vi "Property Dialog.vi"(6 "Control Ref Queue":T15, 7 "Multiplot Representation":T12, 8 "error in (no error)":errorcluster, 11 "2D Error Bar.lvclass in":refnum<class "2D Error Bar.lvclass">) -> (0 "error out":errorcluster, 3 "2D Error Bar.lvclass out":refnum<class "2D Error Bar.lvclass">, 4 "Cancel?":bool)   [LabVIEW 2020, in "2D Error Bar.lvclass"]
uses:
  <vilib>/Math Plots/2D Math Plots/2D Error Bar/2D Error Bar/2D Error Bar.lvclass
  e:/builds/penguin/labview/branches/2020/dev/dist/vi.lib/Math Plots/2D Math Plots/2D Plot/2D Plot/2D Plot.lvclass
  <vilib>/Math Plots/2D Math Plots/2D Plot/Action String/2DMathPlot Ctrl Act Queue.ctl
  <vilib>/Math Plots/2D Math Plots/2D Plot/Action String/2DMathPlot Ctrl Act Cluster.ctl
  <vilib>/Math Plots/2D Math Plots/2D Plot/Action String/2DMathPlot State Class.ctl
  <vilib>/Math Plots/2D Math Plots/2D Plot/2D Plot/Typedef/Multiplot Representation.ctl
  <vilib>/Math Plots/2D Math Plots/2D Plot/2D Plot/Typedef/Plot Representation.ctl
  <vilib>/Math Plots/2D Math Plots/2D Plot/2D Plot/Typedef/Range Cluster.ctl
  <vilib>/Math Plots/2D Math Plots/2D Plot/2D Plot/Typedef/Cursor Property.ctl
  <vilib>/Utility/miscctls.llb/LVCursorListTypeDef.ctl
  <vilib>/Math Plots/2D Math Plots/2D Plot/2D Plot/Typedef/Scale Cluster.ctl
  <vilib>/Utility/miscctls.llb/LVOffsetAndMultiplierTypeDef.ctl
  <vilib>/Math Plots/2D Math Plots/2D Error Bar/2D Error Bar/Typedef/2D Error Bar Property Cluster.ctl
  <vilib>/Math Plots/2D Math Plots/2D Plot/2D Plot/Typedef/Plot Property Array.ctl
  <vilib>/Math Plots/2D Math Plots/2D Plot/2D Plot/Typedef/Plot Property.ctl
  <vilib>/Math Plots/2D Math Plots/2D Error Bar/2D Error Bar/Typedef/2D Error Bar Property Array.ctl
  <vilib>/Math Plots/2D Math Plots/2D Error Bar/2D Error Bar/Typedef/2D Error Bar Property.ctl
  <vilib>/Math Plots/2D Math Plots/2D Plot/2D Plot/Typedef/Graph General Property.ctl
  <vilib>/Math Plots/2D Math Plots/2D Plot/2D Plot/Typedef/Temp Graph Data Action.ctl
  <vilib>/Math Plots/2D Math Plots/2D Plot/2D Plot/Typedef/Temp Graph State.ctl
  <vilib>/Math Plots/2D Math Plots/2D Error Bar/2D Error Bar/2D Error Bar.lvclass/2D Error Bar.ctl
  <vilib>/Math Plots/2D Math Plots/2D Plot/2D Plot/2D Plot.lvclass
panel:
  in  "Graph General":T1
  in  "Format String":string[](array[string])
  in  "Error Bar Property":T2
  in  "Scales Array":T7[](array[typedef])
  in  "Cursor Property":T9
  in  "Dialog Tab":enum32{"UI", "Input & Output"}(tab)
  in  "OK":bool
  in  "Cancel":bool
  in  "Help":bool
  in  "Page Tab":T11(tab)
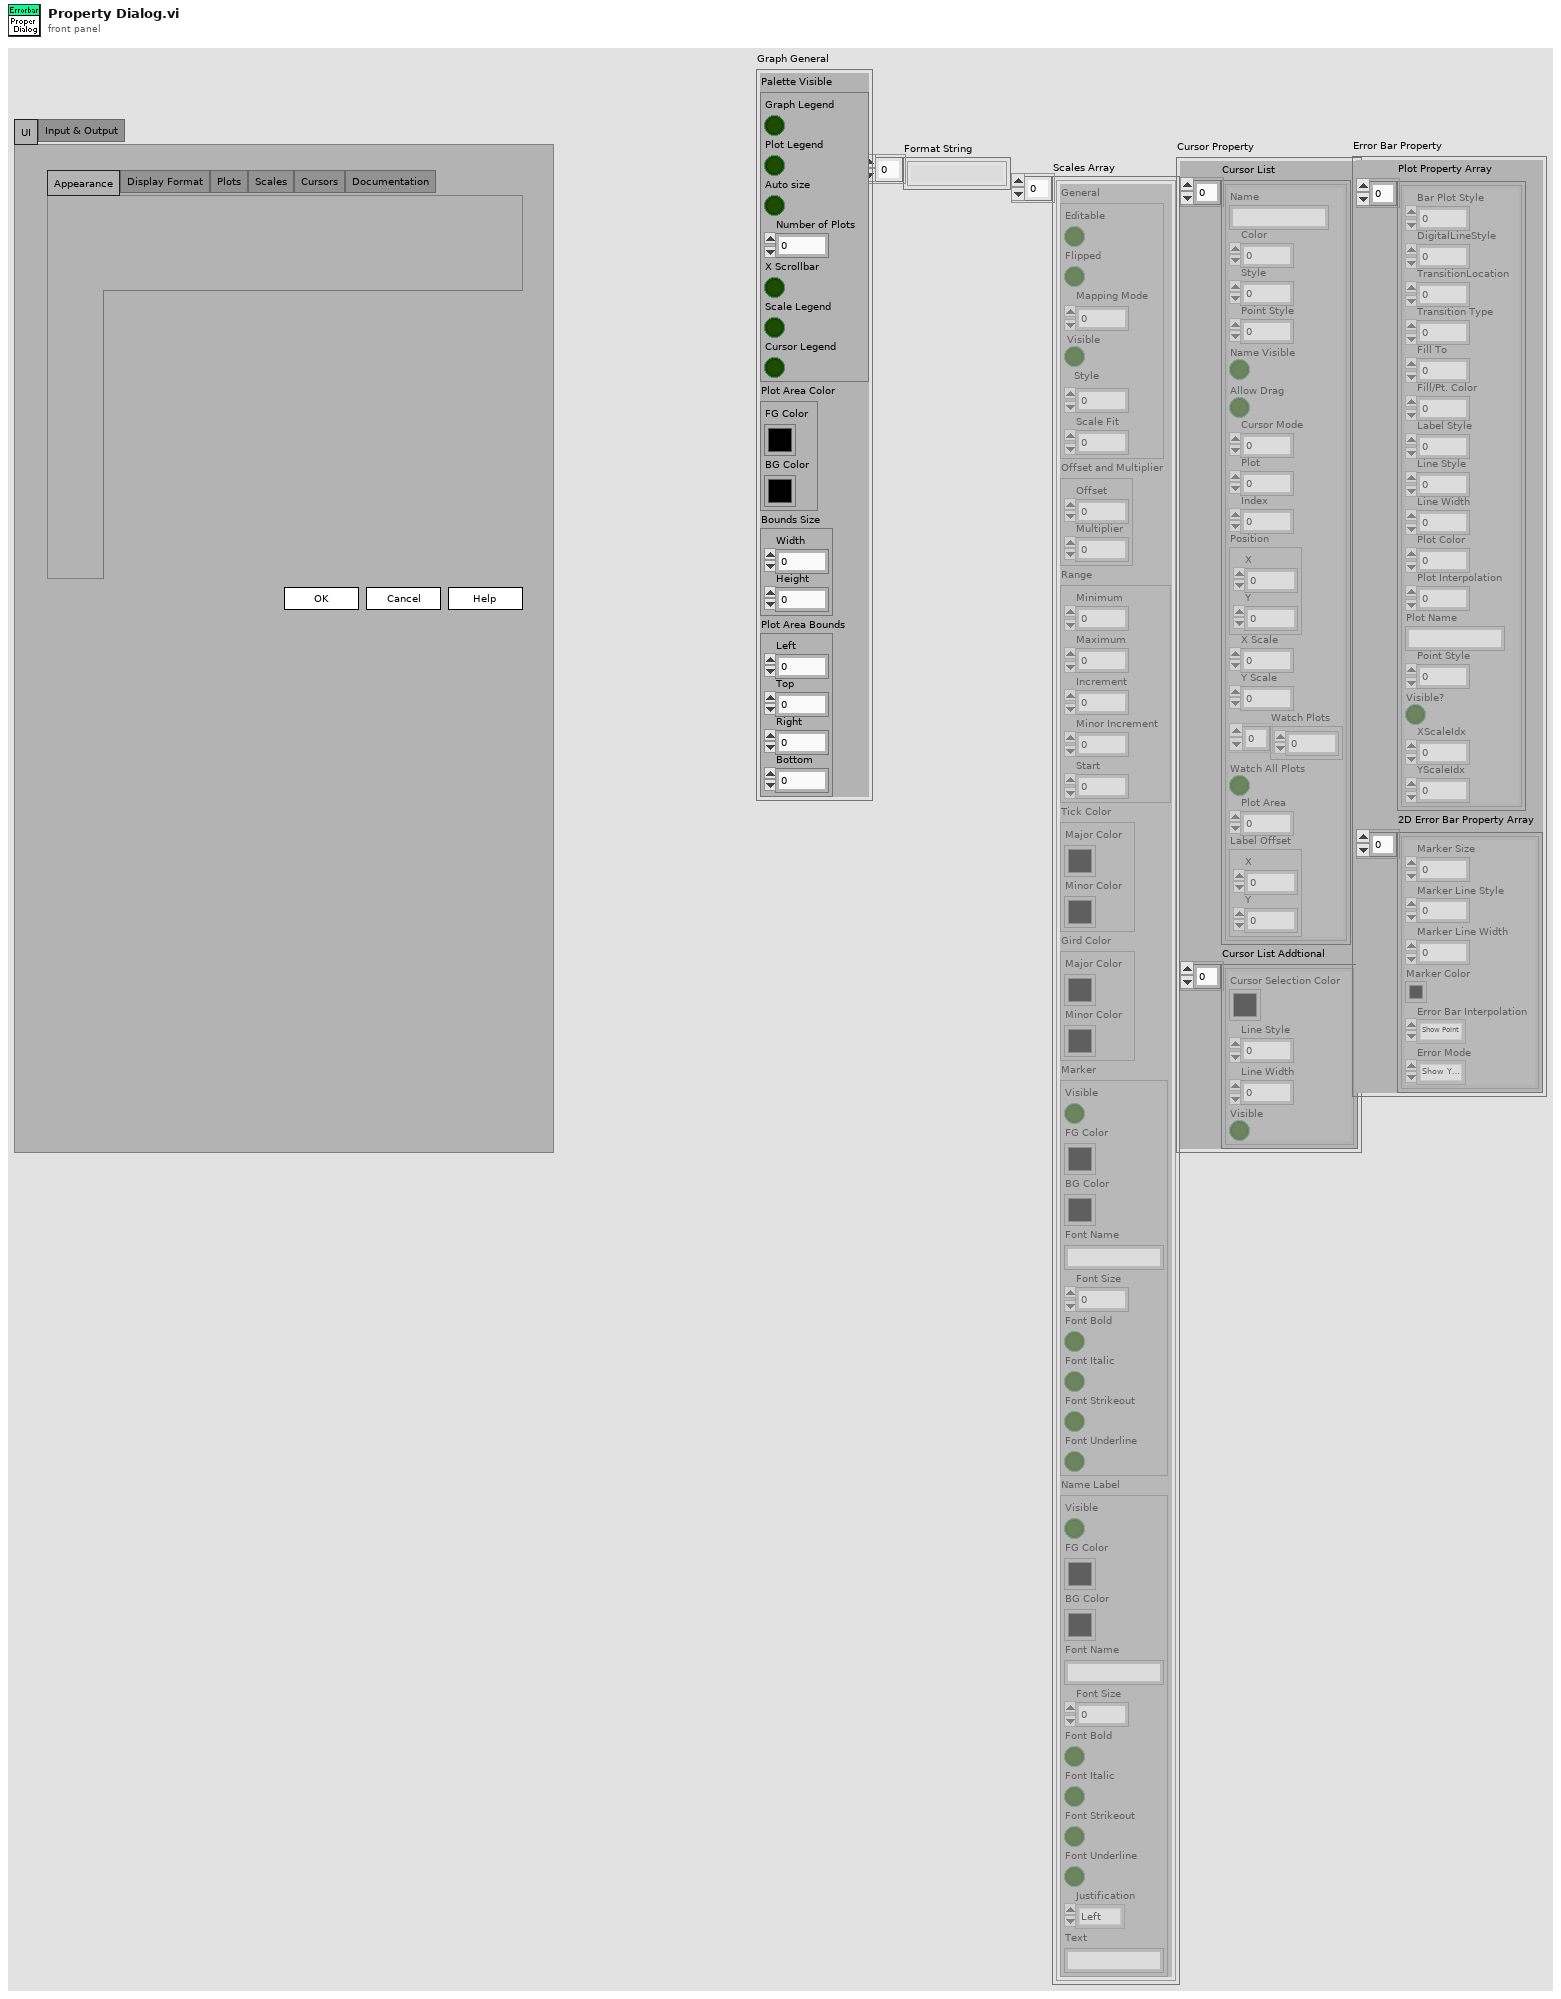
[diagram p1: front panel]
types:
  T1 = typedef "2D Plot.lvclass/Graph General Property.ctl" = cluster{"Palette Visible":cluster{"Graph Legend":bool, "Plot Legend":bool, "Auto size":bool, "Number of Plots":u32, "X Scrollbar":bool, "Scale Legend":bool, "Cursor Legend":bool}, "Plot Area Color":cluster{"FG Color":u32, "BG Color":u32}, "Bounds Size":cluster{"Width":u32, "Height":u32}, "Plot Area Bounds":cluster{"Left":i16, "Top":i16, "Right":i16, "Bottom":i16}}
  T2 = typedef "2D Error Bar.lvclass/2D Error Bar Property Cluster.ctl" = cluster{"Plot Property Array":T3, "2D Error Bar Property Array":T5}
  T3 = typedef "2D Plot.lvclass/Plot Property Array.ctl" = T4[]
  T4 = typedef "2D Plot.lvclass/Plot Property.ctl" = cluster{"Bar Plot Style":u8, "DigitalLineStyle":u8, "TransitionLocation":u8, "Transition Type":u8, "Fill To":i16, "Fill/Pt. Color":u32, "Label Style":u8, "Line Style":u8, "Line Width":u8, "Plot Color":u32, "Plot Interpolation":u8, "Plot Name":string, "Point Style":u8, "Visible?":bool, "XScaleIdx":u32, "YScaleIdx":u32}
  T5 = typedef "2D Error Bar.lvclass/2D Error Bar Property Array.ctl" = T6[]
  T6 = typedef "2D Error Bar.lvclass/2D Error Bar Property.ctl" = cluster{"Marker Size":dbl, "Marker Line Style":u8, "Marker Line Width":u8, "Marker Color":u32, "Error Bar Interpolation":enum16{"Show Point", "Show Line", "Show Bar"}, "Error Mode":enum16{"Show Y Error", "Show X Error", "Show Both Error"}}
  T7 = typedef "2D Plot.lvclass/Scale Cluster.ctl" = cluster{"General":cluster{"Editable":bool, "Flipped":bool, "Mapping Mode":u8, "Visible":bool, "Style":u8, "Scale Fit":u8}, "Offset and Multiplier":T8, "Range":cluster{"Minimum":dbl, "Maximum":dbl, "Increment":dbl, "Minor Increment":dbl, "Start":dbl}, "Tick Color":cluster{"Major Color":u32, "Minor Color":u32}, "Gird Color":cluster{"Major Color":u32, "Minor Color":u32}, "Marker":cluster{"Visible":bool, "FG Color":u32, "BG Color":u32, "Font Name":string, "Font Size":u32, "Font Bold":bool, "Font Italic":bool, "Font Strikeout":bool, "Font Underline":bool}, "Name Label":cluster{"Visible":bool, "FG Color":u32, "BG Color":u32, "Font Name":string, "Font Size":u32, "Font Bold":bool, "Font Italic":bool, "Font Strikeout":bool, "Font Underline":bool, "Justification":enum16{"Left", "Center", "Right"}, "Text":string}}
  T8 = typedef "LVOffsetAndMultiplierTypeDef.ctl" = cluster{"Offset":dbl, "Multiplier":dbl}
  T9 = typedef "2D Plot.lvclass/Cursor Property.ctl" = cluster{"Cursor List":T10, "Cursor List Addtional":cluster{"Cursor Selection Color":u32, "Line Style":u8, "Line Width":u8, "Visible":bool}[]}
  T10 = typedef "LVCursorListTypeDef.ctl" = cluster{"Name":string, "Color":u32, "Style":u8, "Point Style":u8, "Name Visible":bool, "Allow Drag":bool, "Cursor Mode":u32, "Plot":i32, "Index":i32, "Position":cluster{"X":dbl, "Y":dbl}, "X Scale":u32, "Y Scale":u32, "Watch Plots":i32[], "Watch All Plots":bool, "Plot Area":i32, "Label Offset":cluster{"X":dbl, "Y":dbl}}[]
  T11 = enum32{"Appearance", "Display Format", "Plots", "Scales", "Cursors", "Documentation"}
  T12 = typedef "2D Plot.lvclass/Multiplot Representation.ctl" = cluster{"Plot Representation Array":T13[], "Max Range":T14}
  T13 = typedef "2D Plot.lvclass/Plot Representation.ctl" = cluster{"Plot Range":T14, "Vertex Cluster":cluster{"Vertex X Array":dbl[], "Vertex Y Array":dbl[]}, "Base Cluster":cluster{"Base X Array":dbl[], "Base Y Array":dbl[]}}
  T14 = typedef "2D Plot.lvclass/Range Cluster.ctl" = cluster{"X Range":cluster{"Max X":dbl, "Min X":dbl}, "Y Range":cluster{"Max Y":dbl, "Min Y":dbl}}
  T15 = typedef "2DMathPlot Ctrl Act Queue.ctl" = refnum<queue>
  T16 = typedef "2D Plot.lvclass/Temp Graph State.ctl" = enum16{"Create", "Update Graph", "Update Property Only", "Get Plot Name", "Get Axis Name", "Destory"}
  T17 = typedef "2D Plot.lvclass/Temp Graph Data Action.ctl" = enum16{"Data Cluster", "Property Class", "Control Queue"}
  T18 = typedef "2D Plot.lvclass/Property Cluster.ctl" = cluster{"Graph General":T1, "Format Property":string[], "Scale Array":T19, "Cursor Property":T9, "Annotation List":T20, "Active Cursor":i32, "Active Plot":i32}
  T19 = typedef "2D Plot.lvclass/Scale Array.ctl" = T7[]
  T20 = typedef "LVAnnotationListTypeDef.ctl" = cluster{"Name":string, "Color":u32, "Style":u8, "Point Style":u8, "Name Visible":bool, "Allow Drag":bool, "Annotation Mode":u32, "Plot":i32, "Index":i32, "Position":cluster{"X":dbl, "Y":dbl}, "X Scale":u32, "Y Scale":u32, "Show Arrow":bool, "Lock Name":bool, "Plot Area":i32, "Label Offset":cluster{"X":dbl, "Y":dbl}}[]
  T21 = typedef "2DMathPlot Ctrl Act Cluster.ctl" = cluster{"Plot Area Ref":refnum<vi>, "Z Axis Ref":refnum<vi>, "Legend Ref":refnum<vi>, "XControl Ref":refnum<vi>, "Facade Ref":refnum<vi>, "Display State Change Class":T22}
  T22 = typedef "2DMathPlot State Class.ctl" = enum16{"Update All (Undo)", "Update General", "Update Appearance", "Update Format", "Update Scale", "Update Marker", "Update Cursor", "None"}
  T23 = enum8{"Enabled", "Disabled", "Disabled and Grayed Out"}
  T24 = enum32{"Bad", "Idle", "Run top level", "Running"}[]
  T25 = enum32{"Bad", "Idle", "Run top level", "Running"}
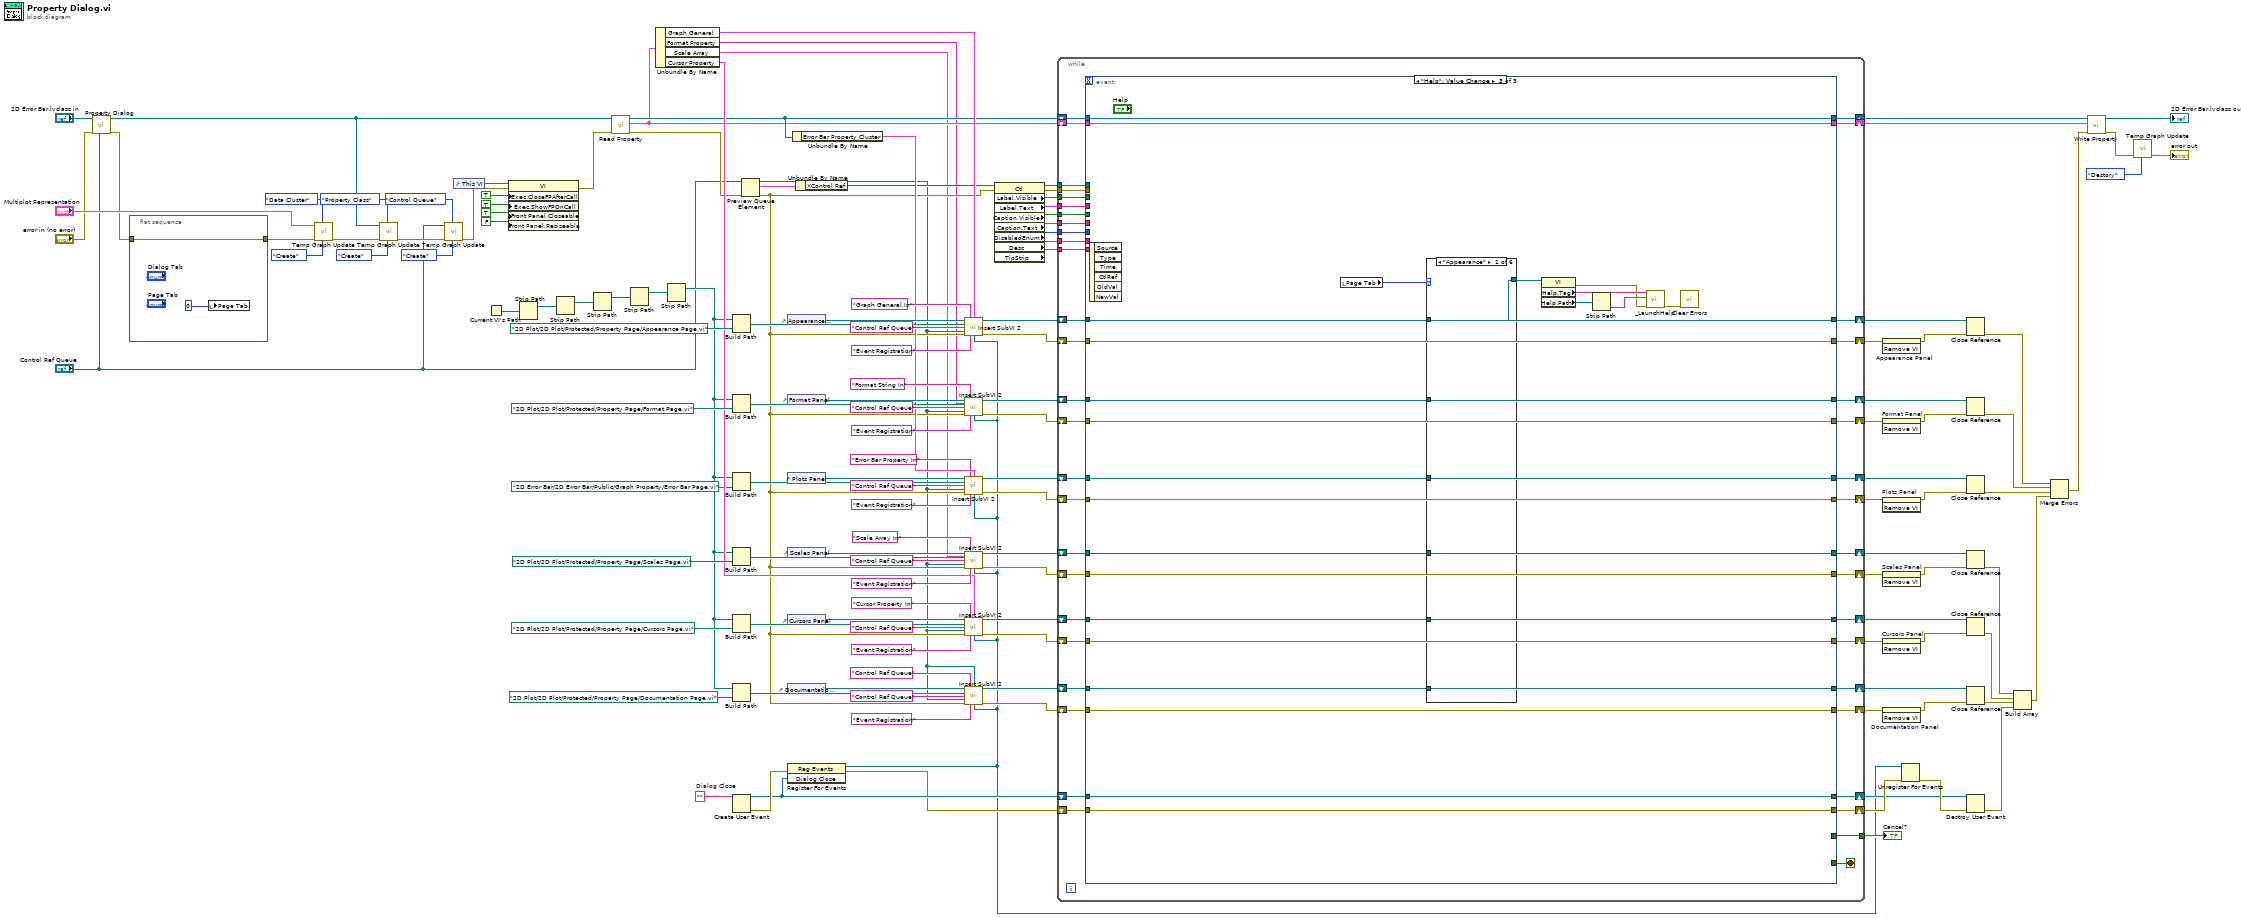
[diagram p0: block diagram]
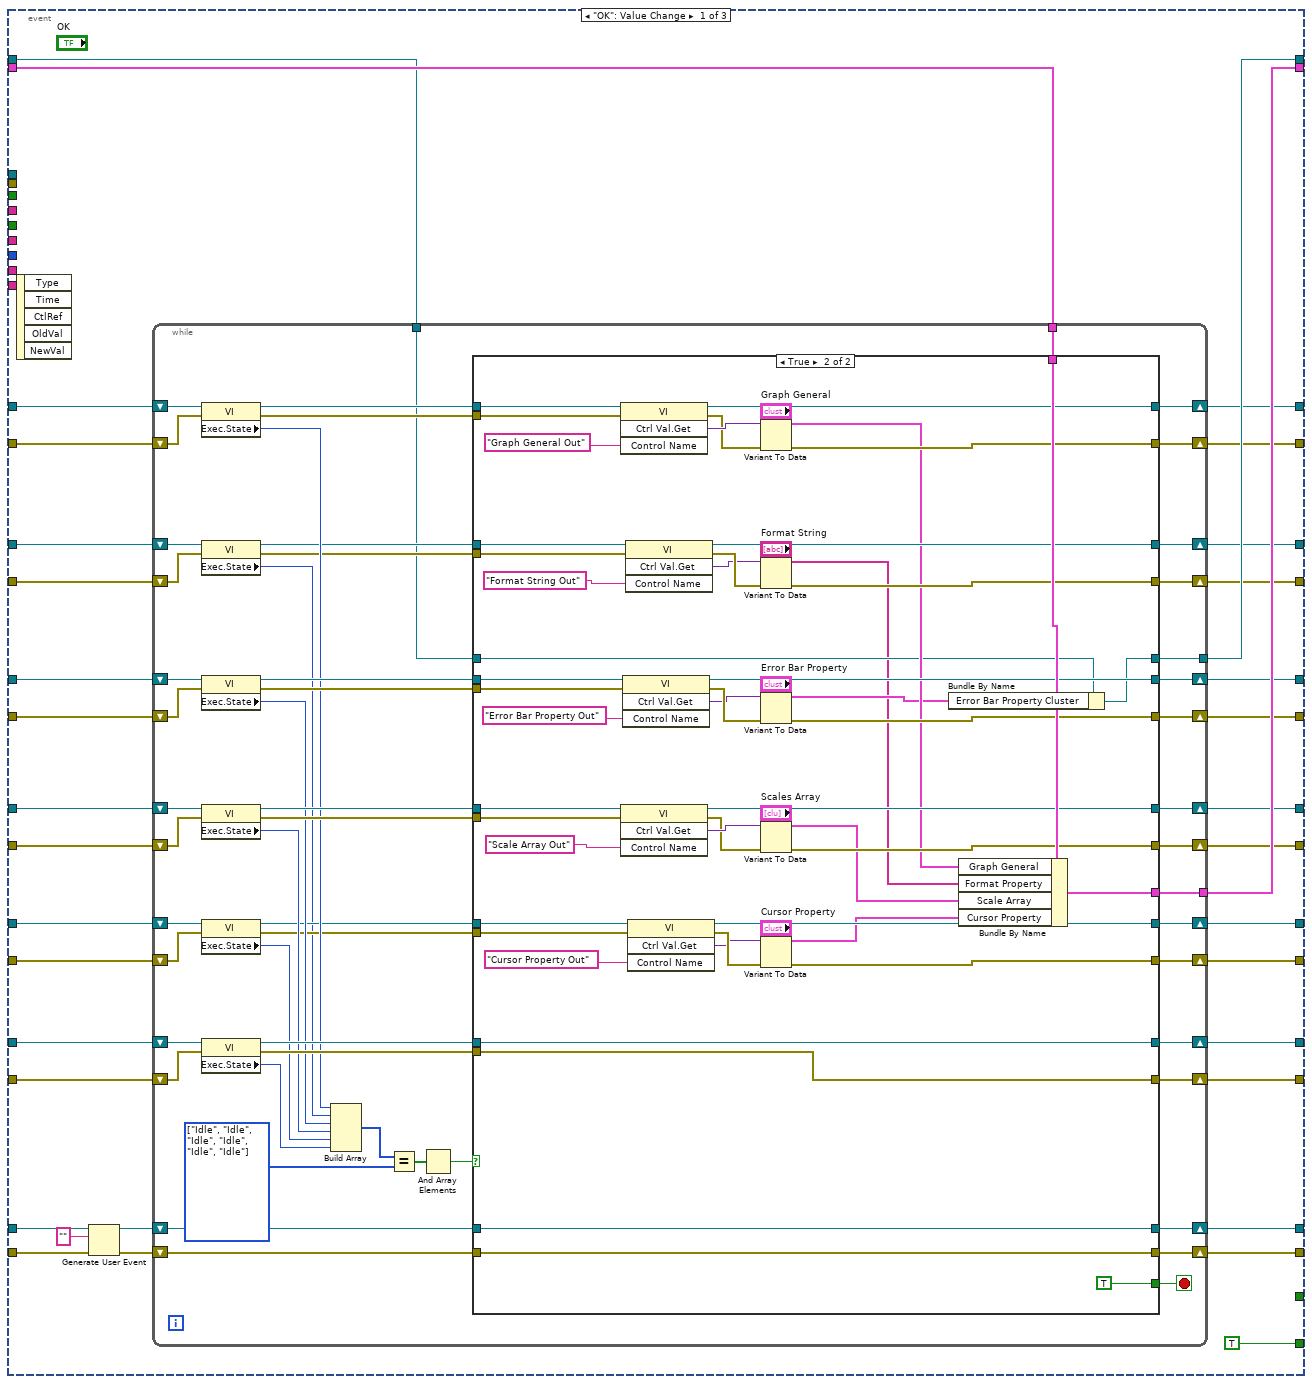
[diagram p2: hidden frame]
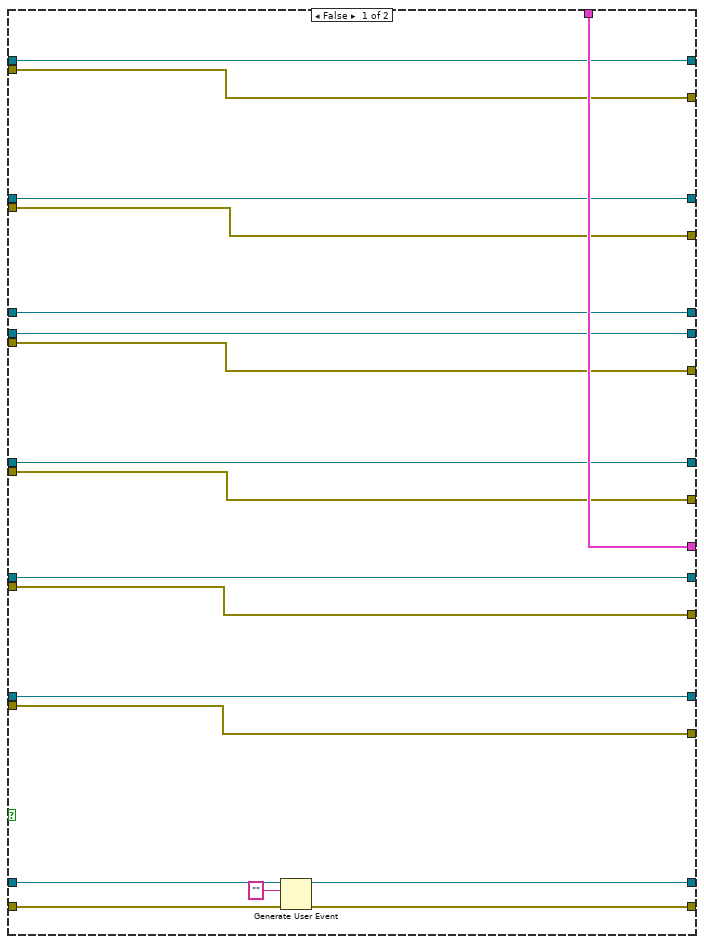
[diagram p3: hidden frame]
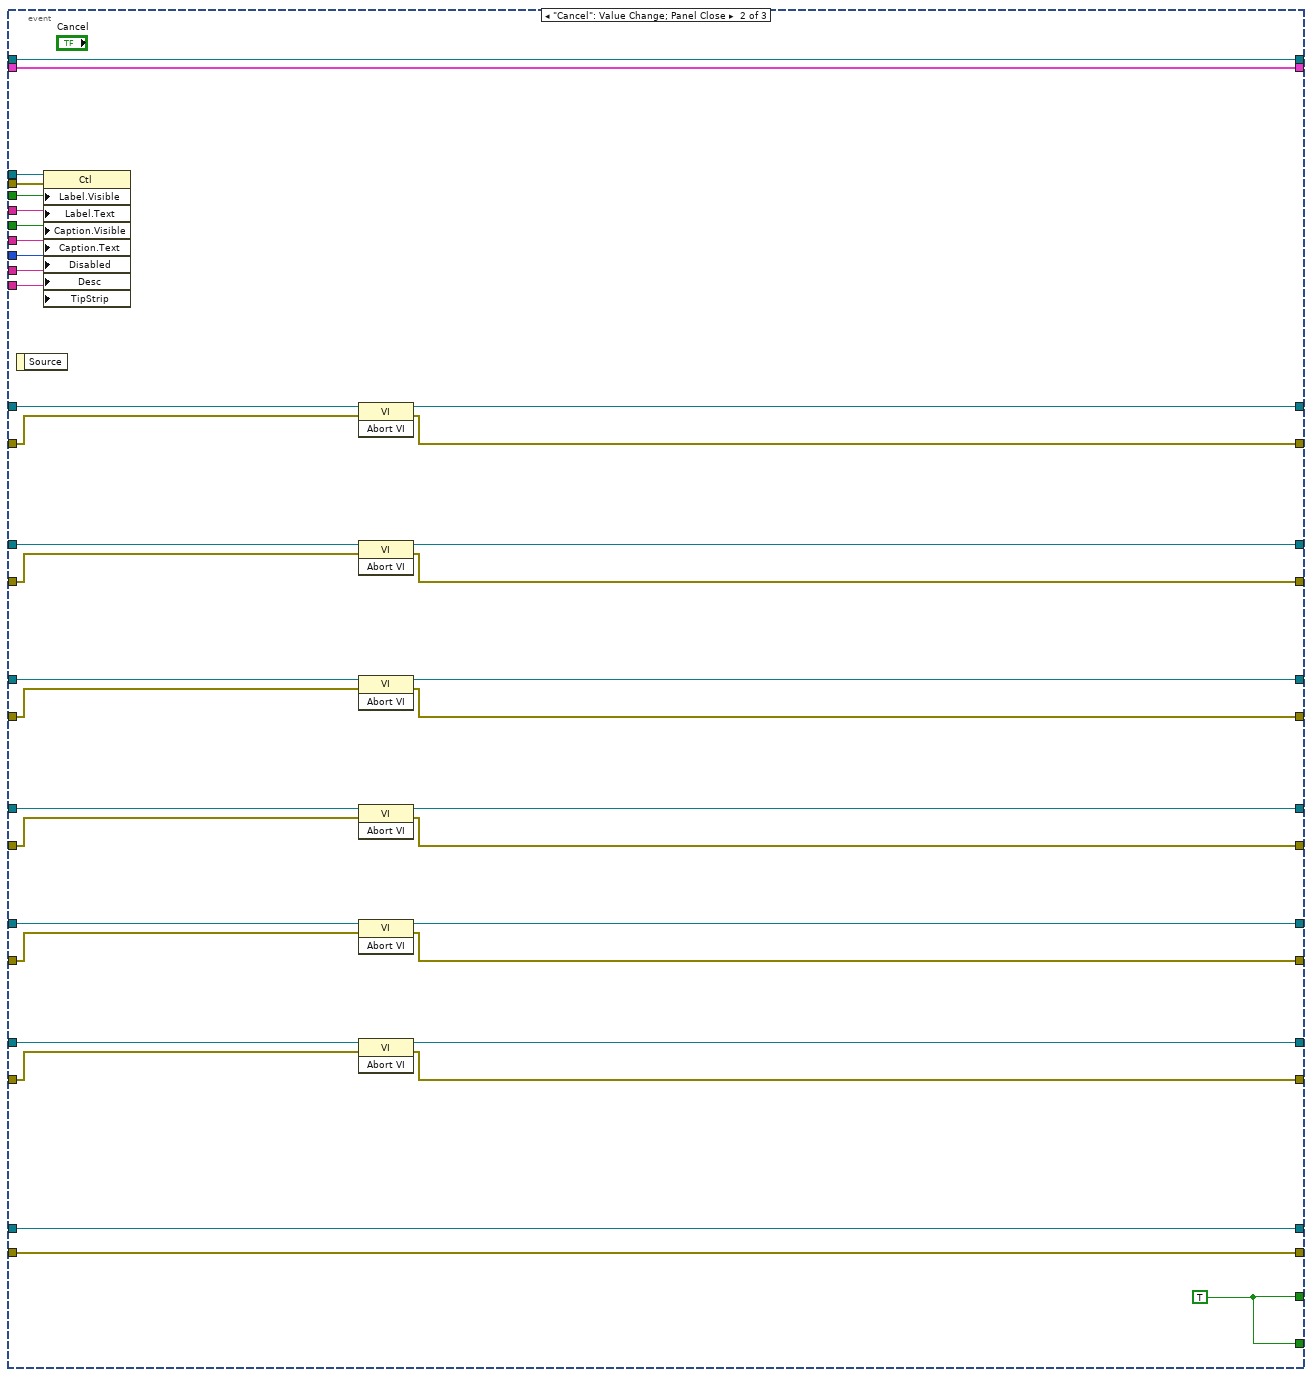
[diagram p4: hidden frame]
diagram:
  w122 = ""  # Dialog Close
  n1 = call-parent "Property Dialog.vi"("Control Ref Queue"="Control Ref Queue", "error in (no error)"="error in (no error)", "2D Plot.lvclass in"="2D Error Bar.lvclass in") -> ("error out"=w2:errorcluster, "2D Plot.lvclass out"=w4:refnum<class "2D Error Bar.lvclass">)  [unwired: 1 in, 6 out]
  n2 = flat-sequence {
    tunnel: w2 -> [w140]
    tunnel: [w140] -> w27
    frame #0 {
      n3 = local write "Page Tab"(u32 0) -> ()
    }
  }
  n4 = call <vilib>:"Temp Graph Update.vi"("State"=Temp_Graph_State."Create", "Data Name"=Temp_Graph_Data_Action."Data Cluster", "error in (no error)"=w27, "Property In"="Multiplot Representation") -> ("error out"=w26:errorcluster)  [unwired: 1 in, 6 out]
  n5 = call <vilib>:"Temp Graph Update.vi"("State"=Temp_Graph_State."Create", "Data Name"=Temp_Graph_Data_Action."Property Class", "error in (no error)"=w26, "Property In"=w4) -> ("error out"=w25:errorcluster)  [unwired: 1 in, 6 out]
  n6 = call <vilib>:"Temp Graph Update.vi"("State"=Temp_Graph_State."Create", "Data Name"=Temp_Graph_Data_Action."Control Queue", "error in (no error)"=w25, "Property In"="Control Ref Queue") -> ("error out"=w18:errorcluster)  [unwired: 1 in, 6 out]
  n7 = control-ref of="This VI"() -> (w139:refnum<vi>)
  n8 = Current VI's Path() -> (path=w131:path)
  n9 = property class="VI"(reference=w139, error in=w18, "Exec.CloseFPAfterCall"=TRUE ("Execution:Close After Call"), "Exec.ShowFPOnCall"=TRUE ("Execution:Show Front Panel On Call"), "Front Panel.Closeable"=TRUE ("Front Panel Window:Closeable"), "Front Panel.Resizeable"=FALSE ("Front Panel Window:Resizeable")) -> (error out=w129:errorcluster)  [unwired: 1 out]
  n10 = Strip Path(path=w131) -> (stripped path=w132:path)  [unwired: 1 out]
  n11 = Strip Path(path=w132) -> (stripped path=w133:path)  [unwired: 1 out]
  n12 = Strip Path(path=w133) -> (stripped path=w130:path)  [unwired: 1 out]
  n13 = call <vilib>:"Read Property.vi"("error in (no error)"=w129, "2D Plot.lvclass in"=w4) -> ("error out"=w39:errorcluster, "XY Graph Property Cluster"=w87:T18, "2D Plot.lvclass out"=w88:refnum<class "2D Error Bar.lvclass">)  [unwired: 7 out]
  n14 = Strip Path(path=w130) -> (stripped path=w7:path)  [unwired: 1 out]
  n15 = Unbundle By Name(w87) -> ("Graph General"=w125:T1, "Format Property"=w9:string[], "Scale Array"=w8:T19, "Cursor Property"=w107:T9)
  n16 = Strip Path(path=w7) -> (stripped path=w6:path)  [unwired: 1 out]
  n17 = Build Path(base path=w6, name or relative path=path "2D Plot/2D Plot/Protected/Property Page/Appearance Page.vi") -> (appended path=w128:path)
  n18 = Build Path(base path=w6, name or relative path=path "2D Plot/2D Plot/Protected/Property Page/Format Page.vi") -> (appended path=w118:path)
  n19 = Build Path(base path=w6, name or relative path=path "2D Error Bar/2D Error Bar/Public/Graph Property/Error Bar Page.vi") -> (appended path=w91:path)
  n20 = Build Path(base path=w6, name or relative path=path "2D Plot/2D Plot/Protected/Property Page/Scales Page.vi") -> (appended path=w112:path)
  n21 = Build Path(base path=w6, name or relative path=path "2D Plot/2D Plot/Protected/Property Page/Cursors Page.vi") -> (appended path=w102:path)
  n22 = Build Path(base path=w6, name or relative path=path "2D Plot/2D Plot/Protected/Property Page/Documentation Page.vi") -> (appended path=w93:path)
  n23 = Create User Event(user event datatype=w122) -> (user event=w74:refnum<user-event>, error out=w123:errorcluster)  [unwired: 1 in]
  n24 = Preview Queue Element(queue="Control Ref Queue", error in (no error)=w39) -> (queue out=w12:T15, element=w38:T21, error out=w13:errorcluster)  [unwired: 2 out]
  n25 = control-ref of="Appearance Panel"() -> (w127:refnum<vi>)
  n26 = control-ref of="Format Panel"() -> (w119:refnum<vi>)
  n27 = control-ref of="Plots Panel"() -> (w98:refnum<vi>)
  n28 = control-ref of="Scales Panel"() -> (w114:refnum<vi>)
  n29 = control-ref of="Cursors Panel"() -> (w104:refnum<vi>)
  n30 = control-ref of="Documentation Panel"() -> (w101:refnum<vi>)
  n31 = register-events(error in=w123, w74) -> (reference out=w11:refnum<event-registration>, error out=w73:errorcluster)  [unwired: 1 in]
  n32 = Unbundle By Name(w88) -> ("Error Bar Property Cluster"=w95:T2)
  n33 = Unbundle By Name(w38) -> ("XControl Ref"=w37:refnum<vi>)
  n34 = call <vilib>:"Insert SubVI 2.vi"("Sub Panel Ref"=w127, "Label 1"="Graph General In", "Value 1"=w125, "VI Path"=w128, "Label 3"="Control Ref Queue" ("Label 1"), "Value 3"=w12, "error in (no error)"=w13, "Label 2"="Event Registration", "Value 2"=w11) -> ("vi reference"=w86:refnum<vi>, "error out"=w80:errorcluster)  [unwired: 5 out]
  n35 = call <vilib>:"Insert SubVI 2.vi"("Sub Panel Ref"=w119, "Label 1"="Format String In" ("Label 2"), "Value 1"=w9, "VI Path"=w118, "Label 3"="Control Ref Queue" ("Label 1"), "Value 3"=w12, "error in (no error)"=w13, "Label 2"="Event Registration", "Value 2"=w11) -> ("vi reference"=w85:refnum<vi>, "error out"=w79:errorcluster)  [unwired: 5 out]
  n36 = call <vilib>:"Insert SubVI 2.vi"("Sub Panel Ref"=w98, "Label 1"="Error Bar Property In", "Value 1"=w95, "VI Path"=w91, "Label 3"="Control Ref Queue" ("Label 1"), "Value 3"=w12, "error in (no error)"=w13, "Label 2"="Event Registration", "Value 2"=w11) -> ("vi reference"=w84:refnum<vi>, "error out"=w78:errorcluster)  [unwired: 5 out]
  n37 = call <vilib>:"Insert SubVI 2.vi"("Sub Panel Ref"=w114, "Label 1"="Scale Array In", "Value 1"=w8, "VI Path"=w112, "Label 3"="Control Ref Queue" ("Label 1"), "Value 3"=w12, "error in (no error)"=w13, "Label 2"="Event Registration", "Value 2"=w11) -> ("vi reference"=w83:refnum<vi>, "error out"=w77:errorcluster)  [unwired: 5 out]
  n38 = call <vilib>:"Insert SubVI 2.vi"("Sub Panel Ref"=w104, "Label 1"="Cursor Property In", "Value 1"=w107, "VI Path"=w102, "Label 3"="Control Ref Queue" ("Label 1"), "Value 3"=w12, "error in (no error)"=w13, "Label 2"="Event Registration", "Value 2"=w11) -> ("vi reference"=w82:refnum<vi>, "error out"=w76:errorcluster)  [unwired: 5 out]
  n39 = call <vilib>:"Insert SubVI 2.vi"("Sub Panel Ref"=w101, "Label 1"="Control Ref Queue", "Value 1"=w12, "VI Path"=w93, "Label 3"="Control Ref Queue" ("Label 1"), "Value 3"=w12, "error in (no error)"=w13, "Label 2"="Event Registration", "Value 2"=w11) -> ("vi reference"=w81:refnum<vi>, "error out"=w75:errorcluster)  [unwired: 5 out]
  n40 = property class="Ctl"(reference=w37, error in=w13) -> (reference out=w36:refnum<vi>, error out=w35:errorcluster, "Label.Visible"=w34:bool, "Label.Text"=w33:string, "Caption.Visible"=w32:bool, "Caption.Text"=w31:string, "DisabledEnum"=w30:T23, "Desc"=w29:string, "TipStrip"=w28:string)
  n41 = while {
    shift-right: [w168] -> w70
    shift-left: w88 -> [w184]
    shift-right: [w167] -> w71
    shift-left: w87 -> [w183]
    shift-right: [w166] -> w61
    shift-left: w80 -> [w176]
    shift-right: [w165] -> w59
    shift-left: w79 -> [w175]
    shift-right: [w164] -> w53
    shift-left: w78 -> [w174]
    shift-right: [w163] -> w50
    shift-left: w77 -> [w173]
    shift-right: [w162] -> w49
    shift-left: w76 -> [w172]
    shift-right: [w161] -> w45
    shift-left: w75 -> [w171]
    shift-right: [w160] -> w42
    shift-left: w73 -> [w169]
    shift-right: [w153] -> w40
    shift-left: w74 -> [w170]
    shift-right: [w154] -> w44
    shift-left: w81 -> [w177]
    shift-right: [w155] -> w48
    shift-left: w82 -> [w178]
    shift-right: [w156] -> w52
    shift-left: w83 -> [w179]
    shift-right: [w157] -> w54
    shift-left: w84 -> [w180]
    shift-right: [w158] -> w57
    shift-left: w85 -> [w181]
    shift-right: [w159] -> w62
    shift-left: w86 -> [w182]
    tunnel: [w151] -> w72
    tunnel: w36 -> [w150]
    tunnel: w35 -> [w149]
    tunnel: w34 -> [w148]
    tunnel: w33 -> [w147]
    tunnel: w32 -> [w146]
    tunnel: w31 -> [w145]
    tunnel: w30 -> [w144]
    tunnel: w29 -> [w143]
    tunnel: w28 -> [w142]
    stop <- w152 stop-if-true
    n42 = event shown="[2] \"Help\": Value Change" {
      selector: _ -> [_ _ _]
      dyn-events: _ -> [_ _ _]
      timeout: _ -> [_ _ _]
      tunnel: w184 -> [w202 w359 w400]
      tunnel: w183 -> [w203 w360 w401]
      tunnel: w182 -> [w220 w386 w392]
      tunnel: w181 -> [w219 w382 w391]
      tunnel: w180 -> [w218 w380 w390]
      tunnel: w179 -> [w217 w378 w389]
      tunnel: w178 -> [w216 w376 w388]
      tunnel: w177 -> [w215 w374 w387]
      tunnel: w176 -> [w214 w385 w409]
      tunnel: w175 -> [w213 w381 w408]
      tunnel: w174 -> [w212 w379 w407]
      tunnel: w173 -> [w211 w377 w406]
      tunnel: w172 -> [w210 w375 w405]
      tunnel: w171 -> [w209 w373 w404]
      tunnel: w170 -> [w205 w362 w402]
      tunnel: w169 -> [w206 w361 w403]
      tunnel: [w201 w359 w400] -> w168
      tunnel: [w200 w360 w401] -> w167
      tunnel: [w199 w383 w409] -> w166
      tunnel: [w198 w371 w408] -> w165
      tunnel: [w185 w369 w407] -> w164
      tunnel: [w186 w367 w406] -> w163
      tunnel: [w197 w365 w405] -> w162
      tunnel: [w196 w363 w404] -> w161
      tunnel: [w195 w361 w403] -> w160
      tunnel: [w194 w384 w392] -> w159
      tunnel: [w193 w372 w391] -> w158
      tunnel: [w192 w370 w390] -> w157
      tunnel: [w191 w368 w389] -> w156
      tunnel: [w190 w366 w388] -> w155
      tunnel: [w189 w364 w387] -> w154
      tunnel: [w187 w362 w402] -> w153
      tunnel: [TRUE w349 _] -> w152
      tunnel: [_ w349 _] -> w151
      tunnel: w150 -> [_ w358 _]
      tunnel: w149 -> [_ w357 _]
      tunnel: w148 -> [_ w356 _]
      tunnel: w147 -> [_ w355 _]
      tunnel: w146 -> [_ w354 _]
      tunnel: w145 -> [_ w353 _]
      tunnel: w144 -> [_ w352 _]
      tunnel: w143 -> [_ w351 _]
      tunnel: w142 -> [_ w350 _]
      event "OK": Value Change {
        n43 = event-data() -> ()  [unwired: 6 out]
        n44 = Generate User Event(user event=w205, event data cluster="" ("event data"), error in=w206) -> (user event out=w204:refnum<user-event>, error out=w207:errorcluster)  [unwired: 1 in]
        n45 = while {
          tunnel: w203 -> [w275]
          tunnel: [w274] -> w200
          shift-right: [w241] -> w187
          shift-left: w204 -> [w242]
          shift-right: [w225] -> w195
          shift-left: w207 -> [w234]
          tunnel: w202 -> [w224]
          tunnel: [w223] -> w201
          shift-right: [w252] -> w196
          shift-left: w209 -> [w248]
          shift-right: [w251] -> w189
          shift-left: w215 -> [w247]
          shift-right: [w228] -> w190
          shift-left: w216 -> [w233]
          shift-right: [w229] -> w197
          shift-left: w210 -> [w232]
          shift-right: [w222] -> w186
          shift-left: w211 -> [w256]
          shift-right: [w253] -> w191
          shift-left: w217 -> [w257]
          shift-right: [w259] -> w192
          shift-left: w218 -> [w262]
          shift-right: [w221] -> w185
          shift-left: w212 -> [w258]
          shift-right: [w236] -> w193
          shift-left: w219 -> [w239]
          shift-right: [w235] -> w198
          shift-left: w213 -> [w240]
          shift-right: [w273] -> w194
          shift-left: w220 -> [w271]
          shift-right: [w272] -> w199
          shift-left: w214 -> [w269]
          stop <- w263 stop-if-true
          w266 = T24 [enum."Idle", enum."Idle", enum."Idle", enum."Idle", enum."Idle", enum."Idle"] items=["Bad", "Idle", "Run top level", "Running"]
          n46 = property class="VI"(reference=w271, error in=w269) -> (reference out=w270:refnum<vi>, error out=w268:errorcluster, "Exec.State"=w246:T25)
          n47 = property class="VI"(reference=w239, error in=w240) -> (reference out=w238:refnum<vi>, error out=w237:errorcluster, "Exec.State"=w227:T25)
          n48 = property class="VI"(reference=w262, error in=w258) -> (reference out=w261:refnum<vi>, error out=w260:errorcluster, "Exec.State"=w245:T25)
          n49 = property class="VI"(reference=w257, error in=w256) -> (reference out=w255:refnum<vi>, error out=w254:errorcluster, "Exec.State"=w244:T25)
          n50 = property class="VI"(reference=w233, error in=w232) -> (reference out=w231:refnum<vi>, error out=w230:errorcluster, "Exec.State"=w226:T25)
          n51 = property class="VI"(reference=w247, error in=w248) -> (reference out=w249:refnum<vi>, error out=w250:errorcluster, "Exec.State"=w243:T25)
          n52 = Build Array(w246, w227, w245, w244, w226, w243) -> (w267:T24)
          n53 = Equal?(x=w267, y=w266) -> (x = y?=w265:bool[])
          n54 = And Array Elements(Boolean array=w265) -> (logical AND=w264:bool)
          n55 = case shown="True" w264 {
            tunnel: w275 -> [w294 w348]
            tunnel: [w294 w347] -> w274
            tunnel: [w293 w343] -> w273
            tunnel: [w292 w342] -> w272
            tunnel: w270 -> [w293 w341]
            tunnel: w268 -> [w292 w340]
            tunnel: [_ TRUE] -> w263
            tunnel: w261 -> [w290 w334]
            tunnel: w260 -> [w291 w335]
            tunnel: [w291 w333] -> w221
            tunnel: [w290 w332] -> w259
            tunnel: w255 -> [w288 w328]
            tunnel: w254 -> [w289 w327]
            tunnel: [w288 w326] -> w253
            tunnel: [w289 w325] -> w222
            tunnel: w249 -> [w287 w298]
            tunnel: w250 -> [w286 w297]
            tunnel: [w287 w298] -> w251
            tunnel: [w286 w297] -> w252
            tunnel: w242 -> [w285 w324]
            tunnel: [w284 w324] -> w241
            tunnel: w238 -> [w282 w320]
            tunnel: w237 -> [w281 w319]
            tunnel: [w282 w318] -> w236
            tunnel: [w281 w317] -> w235
            tunnel: w234 -> [w280 w316]
            tunnel: [w279 w316] -> w225
            tunnel: w231 -> [w278 w312]
            tunnel: w230 -> [w277 w311]
            tunnel: [w277 w310] -> w229
            tunnel: [w278 w309] -> w228
            tunnel: w224 -> [w276 w305]
            tunnel: [w276 w299] -> w223
            frame False {
              n56 = Generate User Event(user event=w285, event data cluster="" ("event data"), error in=w280) -> (user event out=w284:refnum<user-event>, error out=w279:errorcluster)  [unwired: 1 in]
            }
            frame True {
              n57 = invoke class="VI" method="Ctrl Val.Get"(reference=w341, error in=w340, "Control Name"="Graph General Out") -> (reference out=w343:refnum<vi>, error out=w344:errorcluster, "Get Control Value Variant"=w345:variant)  [unwired: 1 in, 1 out]
              n58 = invoke class="VI" method="Ctrl Val.Get"(reference=w328, error in=w327, "Control Name"="Scale Array Out") -> (reference out=w326:refnum<vi>, error out=w329:errorcluster, "Get Control Value Variant"=w330:variant)  [unwired: 1 in, 1 out]
              n59 = invoke class="VI" method="Ctrl Val.Get"(reference=w334, error in=w335, "Control Name"="Error Bar Property Out") -> (reference out=w332:refnum<vi>, error out=w338:errorcluster, "Get Control Value Variant"=w337:variant)  [unwired: 1 in, 1 out]
              n60 = invoke class="VI" method="Ctrl Val.Get"(reference=w320, error in=w319, "Control Name"="Format String Out") -> (reference out=w318:refnum<vi>, error out=w323:errorcluster, "Get Control Value Variant"=w322:variant)  [unwired: 1 in, 1 out]
              n61 = invoke class="VI" method="Ctrl Val.Get"(reference=w312, error in=w311, "Control Name"="Cursor Property Out") -> (reference out=w309:refnum<vi>, error out=w315:errorcluster, "Get Control Value Variant"=w314:variant)  [unwired: 1 in, 1 out]
              n62 = Variant To Data(error in=w344, type="Graph General", Variant=w345) -> (data=w307:T1, error out=w342:errorcluster)
              n63 = Variant To Data(error in=w323, type="Format String", Variant=w322) -> (data=w295:string[], error out=w317:errorcluster)
              n64 = Variant To Data(error in=w338, type="Error Bar Property", Variant=w337) -> (data=w303:T2, error out=w333:errorcluster)
              n65 = Variant To Data(error in=w329, type="Scales Array", Variant=w330) -> (data=w296:T7[], error out=w325:errorcluster)
              n66 = Variant To Data(error in=w315, type="Cursor Property", Variant=w314) -> (data=w300:T9, error out=w310:errorcluster)
              n67 = Bundle By Name(cluster=w305, "Error Bar Property Cluster"=w303) -> (w299:refnum<class "2D Error Bar.lvclass">)
              n68 = Bundle By Name(cluster=w348, "Graph General"=w307, "Format Property"=w295, "Scale Array"=w296, "Cursor Property"=w300) -> (w347:T18)
            }
          }
        }
      }
      event "Cancel": Value Change; Panel Close {
        w349 = TRUE
        n69 = event-data() -> ()  [unwired: 2 out]
        n70 = property class="Ctl"(reference=w358, error in=w357, "Label.Visible"=w356, "Label.Text"=w355, "Caption.Visible"=w354, "Caption.Text"=w353, "Disabled"=w352, "Desc"=w351, "TipStrip"=w350) -> ()  [unwired: 2 out]
        n71 = invoke class="VI" method="Abort VI"(reference=w386, error in=w385) -> (reference out=w384:refnum<vi>, error out=w383:errorcluster)  [unwired: 1 in, 1 out]
        n72 = invoke class="VI" method="Abort VI"(reference=w382, error in=w381) -> (reference out=w372:refnum<vi>, error out=w371:errorcluster)  [unwired: 1 in, 1 out]
        n73 = invoke class="VI" method="Abort VI"(reference=w380, error in=w379) -> (reference out=w370:refnum<vi>, error out=w369:errorcluster)  [unwired: 1 in, 1 out]
        n74 = invoke class="VI" method="Abort VI"(reference=w378, error in=w377) -> (reference out=w368:refnum<vi>, error out=w367:errorcluster)  [unwired: 1 in, 1 out]
        n75 = invoke class="VI" method="Abort VI"(reference=w376, error in=w375) -> (reference out=w366:refnum<vi>, error out=w365:errorcluster)  [unwired: 1 in, 1 out]
        n76 = invoke class="VI" method="Abort VI"(reference=w374, error in=w373) -> (reference out=w364:refnum<vi>, error out=w363:errorcluster)  [unwired: 1 in, 1 out]
      }
      event "Help": Value Change {
        n77 = event-data() -> ()  [unwired: 7 out]
        n78 = local read "Page Tab"() -> (w393:T11)
        n79 = case shown="\"Appearance\"" w393 {
          tunnel: w392 -> [w410 _ _ _ _ _]
          tunnel: [w410 w411 w412 w413 w414 w415] -> w394
          tunnel: w391 -> [_ w411 _ _ _ _]
          tunnel: w390 -> [_ _ w412 _ _ _]
          tunnel: w389 -> [_ _ _ w413 _ _]
          tunnel: w388 -> [_ _ _ _ w414 _]
          tunnel: w387 -> [_ _ _ _ _ w415]
          frame "Appearance" {
          }
          frame "Display Format" {
          }
          frame "Plots" {
          }
          frame "Scales" {
          }
          frame "Cursors" {
          }
          frame "Documentation" {
          }
        }
        n80 = property class="VI"(reference=w394) -> (error out=w396:errorcluster, "Help.Tag"=w398:string, "Help.Path"=w399:path)  [unwired: 1 in, 1 out]
        n81 = Strip Path(path=w399) -> (name=w397:string)  [unwired: 1 out]
        n82 = call <helpdir>:"_LaunchHelp.vi"("error in (no error)"=w396, "CHM or HLP filename (lvdialog.chm)"=w397, "HTML filename"=w398) -> ("error out"=w395:errorcluster)  [unwired: 4 out]
        n83 = call <vilib>:"Clear Errors.vi"("error in (no error)"=w395) -> ()  [unwired: 5 in, 2 out]
      }
    }
  }
  "Cancel?" <- w72
  n84 = invoke on="Appearance Panel" class="SubPnl" method="Remove VI"(error in=w61) -> (error out=w60:errorcluster)  [unwired: 2 in, 2 out]
  n85 = invoke on="Format Panel" class="SubPnl" method="Remove VI"(error in=w59) -> (error out=w58:errorcluster)  [unwired: 2 in, 2 out]
  n86 = invoke on="Plots Panel" class="SubPnl" method="Remove VI"(error in=w53) -> (error out=w55:errorcluster)  [unwired: 2 in, 2 out]
  n87 = invoke on="Scales Panel" class="SubPnl" method="Remove VI"(error in=w50) -> (error out=w51:errorcluster)  [unwired: 2 in, 2 out]
  n88 = invoke on="Cursors Panel" class="SubPnl" method="Remove VI"(error in=w49) -> (error out=w47:errorcluster)  [unwired: 2 in, 2 out]
  n89 = invoke on="Documentation Panel" class="SubPnl" method="Remove VI"(error in=w45) -> (error out=w46:errorcluster)  [unwired: 2 in, 2 out]
  n90 = Unregister For Events(event registration refnum=w11, error in=w42) -> (error out=w41:errorcluster)
  n91 = Close Reference(reference=w62, error in (no error)=w60) -> (error out=w56:errorcluster)
  n92 = Close Reference(reference=w57, error in (no error)=w58) -> (error out=w66:errorcluster)
  n93 = Close Reference(reference=w54, error in (no error)=w55) -> (error out=w65:errorcluster)
  n94 = Close Reference(reference=w52, error in (no error)=w51) -> (error out=w67:errorcluster)
  n95 = Close Reference(reference=w48, error in (no error)=w47) -> (error out=w68:errorcluster)
  n96 = Close Reference(reference=w44, error in (no error)=w46) -> (error out=w63:errorcluster)
  n97 = Destroy User Event(user event=w40, error in=w41) -> (error out=w10:errorcluster)
  n98 = Build Array(w67, w68, w63, w10) -> (w64:errorcluster[])
  n99 = Merge Errors(w56, w66, w65, w64) -> (w43:errorcluster)
  n100 = call <vilib>:"Write Property.vi"("error in (no error)"=w43, "XY Graph Property Cluster"=w71, "2D Plot.lvclass in"=w70) -> ("error out"=w17:errorcluster, "2D Plot.lvclass out"=→"2D Error Bar.lvclass out":refnum<class "2D Error Bar.lvclass">)  [unwired: 7 out]
  n101 = call <vilib>:"Temp Graph Update.vi"("State"=Temp_Graph_State."Destory", "error in (no error)"=w17) -> ("error out"=→"error out":errorcluster)  [unwired: 3 in, 6 out]
